vi "CR-Initial CameraCCD345.vi"(8 "error in (no error)":errorcluster caption="错误输入（无错误）") -> (0 "error out":errorcluster caption="错误输出", 1 "Session Out5":T1, 2 "Session Out6":T1, 3 "Session Out4":T1)   [LabVIEW 2017]
uses:
  <vilib>/userdefined/High Color/IMAQdx.ctl
  <vilib>/vision/driver/IMAQdx.llb/IMAQdx Camera Control Mode.ctl
  <vilib>/vision/driver/IMAQdx.llb/IMAQdx Acquisition Mode.ctl
  <vilib>/vision/driver/NI_Vision_Acquisition_Software.lvlib
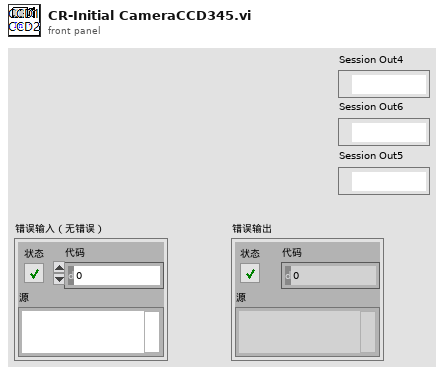
[diagram p1: front panel]
types:
  T1 = typedef "IMAQdx.ctl" = refnum<k21>
  T2 = typedef "NI_Vision_Acquisition_Software.lvlib/IMAQdx Acquisition Mode.ctl" = enum32{"One Shot", "Continuous"}
  T3 = typedef "NI_Vision_Acquisition_Software.lvlib/IMAQdx Camera Control Mode.ctl" = enum32{"Controller", "Listener"}
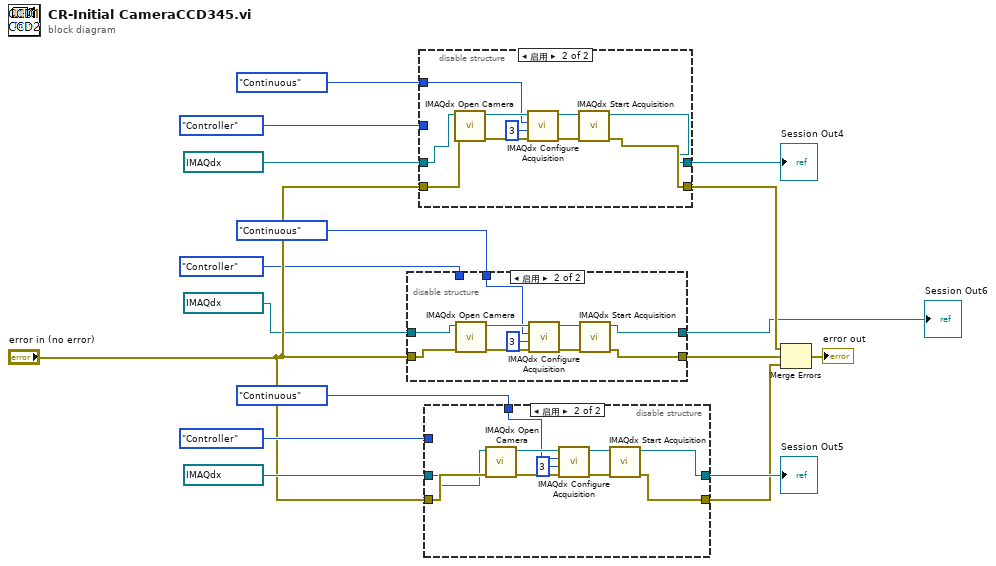
[diagram p0: block diagram]
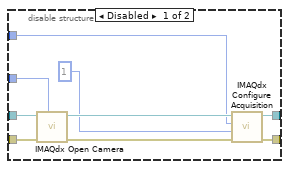
[diagram p2: hidden frame]
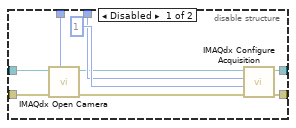
[diagram p3: hidden frame]
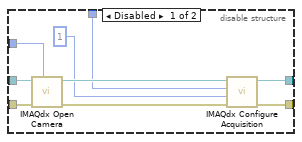
[diagram p4: hidden frame]
diagram:
  n1 = disable-structure shown="启用" {
    disable-tunnel: T1 "cam6" ("Session In") -> [w26 w28]
    disable-tunnel: IMAQdx_Acquisition_Mode."Continuous" ("Continuous?") -> [w23 w27]
    disable-tunnel: IMAQdx_Camera_Control_Mode."Controller" ("Camera Control Mode") -> [w21 _]
    disable-tunnel: [w20 w31] -> w3
    disable-tunnel: [w19 w30] -> w1
    disable-tunnel: "error in (no error)" -> [w18 w29]
    frame Disabled {
      n2 = call <vilib>:"IMAQdx Open Camera.vi"("Camera Control Mode"=w21, "error in"=w18, "Session In"=w26) -> ("error out"=w25:errorcluster, "Session Out"=w22:T1)  [unwired: 7 in]
      n3 = call <vilib>:"IMAQdx Configure Acquisition.vi"("error in"=w25, "Number of Buffers"=u32 1, "Continuous?"=w23, "Session In"=w22) -> ("error out"=w19:errorcluster, "Session Out"=w20:T1)  [unwired: 6 in]
    }
    frame Enabled {
      n4 = call <vilib>:"IMAQdx Open Camera.vi"("error in"=w29, "Session In"=w28) -> ("error out"=w35:errorcluster, "Session Out"=w33:T1)  [unwired: 1 in, 7 out]
      n5 = call <vilib>:"IMAQdx Configure Acquisition.vi"("error in"=w35, "Number of Buffers"=u32 3, "Continuous?"=w27, "Session In"=w33) -> ("error out"=w36:errorcluster, "Session Out"=w34:T1)  [unwired: 6 out]
      n6 = call <vilib>:"IMAQdx Start Acquisition.vi"("error in"=w36, "Session In"=w34) -> ("error out"=w30:errorcluster, "Session Out"=w31:T1)  [unwired: 8 out]
    }
  }
  "Session Out6" <- w3
  n7 = disable-structure shown="启用" {
    disable-tunnel: [w45 w48] -> w11
    disable-tunnel: IMAQdx_Camera_Control_Mode."Controller" ("Camera Control Mode") -> [w44 _]
    disable-tunnel: IMAQdx_Acquisition_Mode."Continuous" ("Continuous?") -> [w42 w46]
    disable-tunnel: T1 "cam4" ("Session In") -> [w39 w50]
    disable-tunnel: [w38 w47] -> w7
    disable-tunnel: "error in (no error)" -> [w37 w49]
    frame Disabled {
      n8 = call <vilib>:"IMAQdx Open Camera.vi"("Camera Control Mode"=w44, "error in"=w37, "Session In"=w39) -> ("error out"=w40:errorcluster, "Session Out"=w43:T1)  [unwired: 7 in]
      n9 = call <vilib>:"IMAQdx Configure Acquisition.vi"("error in"=w40, "Number of Buffers"=u32 1, "Continuous?"=w42, "Session In"=w43) -> ("error out"=w45:errorcluster, "Session Out"=w38:T1)  [unwired: 6 in]
    }
    frame Enabled {
      n10 = call <vilib>:"IMAQdx Open Camera.vi"("error in"=w49, "Session In"=w50) -> ("error out"=w54:errorcluster, "Session Out"=w52:T1)  [unwired: 1 in, 7 out]
      n11 = call <vilib>:"IMAQdx Configure Acquisition.vi"("error in"=w54, "Number of Buffers"=u32 3, "Continuous?"=w46, "Session In"=w52) -> ("error out"=w55:errorcluster, "Session Out"=w53:T1)  [unwired: 6 out]
      n12 = call <vilib>:"IMAQdx Start Acquisition.vi"("error in"=w55, "Session In"=w53) -> ("error out"=w48:errorcluster, "Session Out"=w47:T1)  [unwired: 8 out]
    }
  }
  "Session Out4" <- w7
  n13 = disable-structure shown="启用" {
    disable-tunnel: IMAQdx_Camera_Control_Mode."Controller" ("Camera Control Mode") -> [w64 _]
    disable-tunnel: IMAQdx_Acquisition_Mode."Continuous" ("Continuous?") -> [w62 w66]
    disable-tunnel: T1 "cam5" ("Session In") -> [w59 w67]
    disable-tunnel: [w58 w68] -> w14
    disable-tunnel: "error in (no error)" -> [w57 w70]
    disable-tunnel: [w56 w69] -> w12
    frame Disabled {
      n14 = call <vilib>:"IMAQdx Open Camera.vi"("Camera Control Mode"=w64, "error in"=w57, "Session In"=w59) -> ("error out"=w60:errorcluster, "Session Out"=w63:T1)  [unwired: 7 in]
      n15 = call <vilib>:"IMAQdx Configure Acquisition.vi"("error in"=w60, "Number of Buffers"=u32 1, "Continuous?"=w62, "Session In"=w63) -> ("error out"=w56:errorcluster, "Session Out"=w58:T1)  [unwired: 6 in]
    }
    frame Enabled {
      n16 = call <vilib>:"IMAQdx Open Camera.vi"("error in"=w70, "Session In"=w67) -> ("error out"=w73:errorcluster, "Session Out"=w71:T1)  [unwired: 1 in, 7 out]
      n17 = call <vilib>:"IMAQdx Configure Acquisition.vi"("error in"=w73, "Number of Buffers"=u32 3, "Continuous?"=w66, "Session In"=w71) -> ("error out"=w74:errorcluster, "Session Out"=w72:T1)  [unwired: 6 out]
      n18 = call <vilib>:"IMAQdx Start Acquisition.vi"("error in"=w74, "Session In"=w72) -> ("error out"=w69:errorcluster, "Session Out"=w68:T1)  [unwired: 8 out]
    }
  }
  "Session Out5" <- w14
  n19 = Merge Errors(w11, w1, w12) -> (→"error out":errorcluster)
